vi "Conf Temp.vi"(8 "error in (no error)":errorcluster, 11 "IncTemperature":T1={"ConnectedTempSensor"="100", "ConvertMode"="1", "InitGainSelection"="0", "FrequencySelection"="240", "PowerSaveMode"=FALSE, "GainSelection"="", "RefValue"=0.0}) -> (0 "error out":errorcluster, 3 "IncTemperature Out":T1={"ConnectedTempSensor"="500", "ConvertMode"="1", "InitGainSelection"="32", "FrequencySelection"="240 Hz", "PowerSaveMode"=FALSE, "GainSelection"="", "RefValue"=0.0})   [LabVIEW 2014, in "MSX-E3711_dll.lvlib"]
uses:
  MSX-E3711_dll.lvlib
panel:
  in  "Frecuencia":string(combo)="240 Hz"
  in  "Ganancia":string(combo)="0"
  in  "Unidad":string(combo)="1"
  in  "Tipo de Sensor":string(combo)="1000"
  in  "Cancelar":bool
  in  "Save Button":bool
  # "Configurar Temperatura"
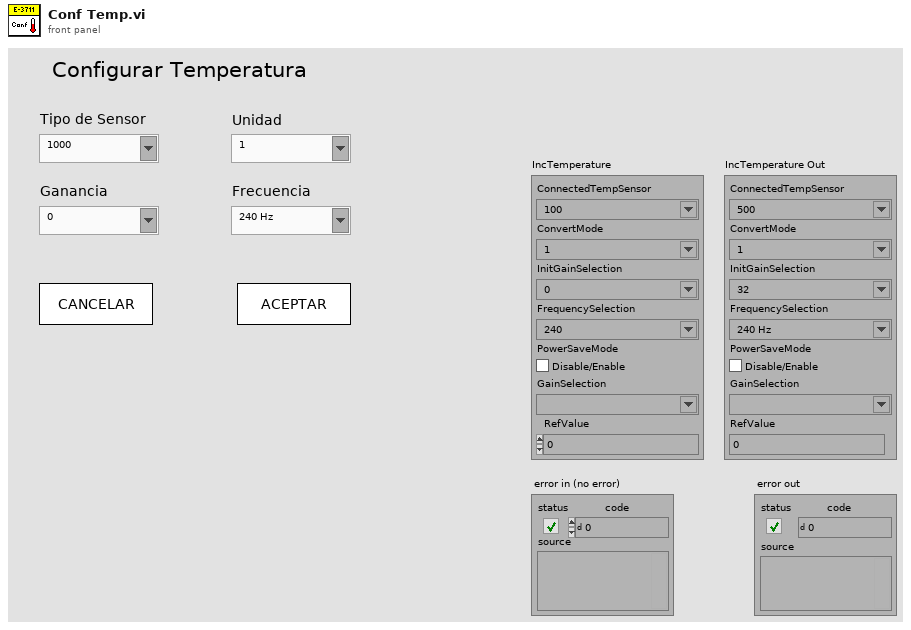
[diagram p1: front panel]
types:
  T1 = cluster{"ConnectedTempSensor":string, "ConvertMode":string, "InitGainSelection":string, "FrequencySelection":string, "PowerSaveMode":bool, "GainSelection":string, "RefValue":dbl}
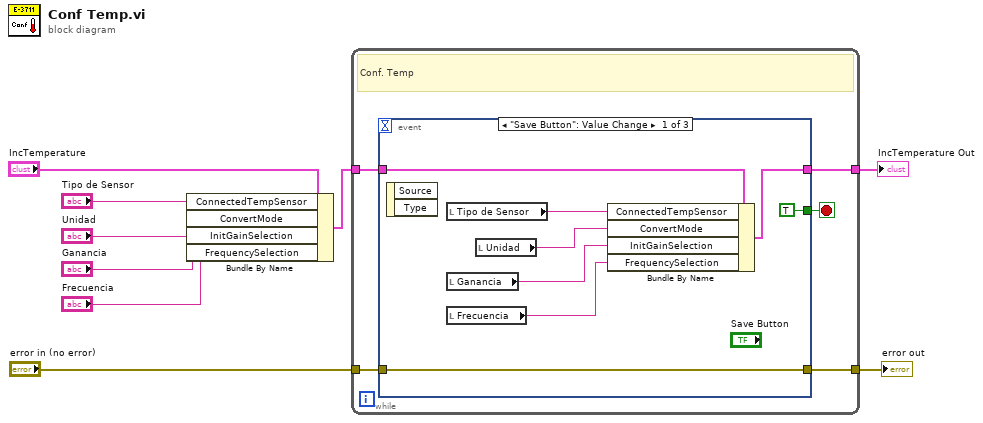
[diagram p0: block diagram]
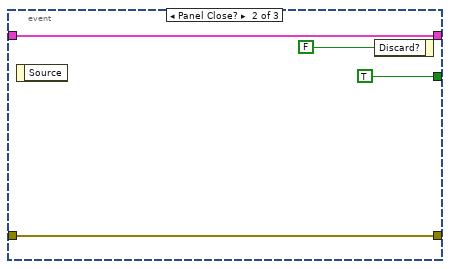
[diagram p2: hidden frame]
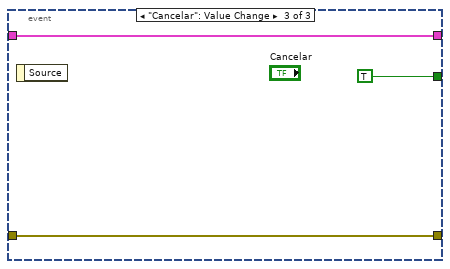
[diagram p3: hidden frame]
diagram:
  n1 = Bundle By Name(cluster="IncTemperature", "ConnectedTempSensor"="Tipo de Sensor", "ConvertMode"="Unidad", "InitGainSelection"="Ganancia", "FrequencySelection"="Frecuencia") -> (w5:T1)
  n2 = while {
    tunnel: [w13] -> w9
    tunnel: w5 -> [w12]
    tunnel: "error in (no error)" -> [w11]
    tunnel: [w10] -> w7
    stop <- w14 stop-if-true
    # "Conf. Temp"
    n3 = event shown="[0] \"Save Button\": Value Change" {
      selector: _ -> [_ _ _]
      dyn-events: _ -> [_ _ _]
      timeout: _ -> [_ _ _]
      tunnel: [TRUE ("Save Button") TRUE ("Save Button") TRUE ("Save Button")] -> w14
      tunnel: [w19 w24 w28] -> w13
      tunnel: w12 -> [w20 w24 w28]
      tunnel: w11 -> [w21 w23 w27]
      tunnel: [w21 w23 w27] -> w10
      event "Save Button": Value Change {
        n4 = event-data() -> ()  [unwired: 1 in, 2 out]
        n5 = local read "Tipo de Sensor"() -> (w18:string)
        n6 = local read "Ganancia"() -> (w16:string)
        n7 = local read "Frecuencia"() -> (w15:string)
        n8 = local read "Unidad"() -> (w17:string)
        n9 = Bundle By Name(cluster=w20, "ConnectedTempSensor"=w18, "ConvertMode"=w17, "InitGainSelection"=w16, "FrequencySelection"=w15) -> (w19:T1)
      }
      event Panel Close? {
        n10 = event-data() -> ()  [unwired: 1 in, 1 out]
        n11 = event-data("Discard?"=FALSE) -> ()  [unwired: 1 in, 1 out]
      }
      event "Cancelar": Value Change {
        n12 = event-data() -> ()  [unwired: 1 in, 1 out]
      }
    }
  }
  "error out" <- w7
  "IncTemperature Out" <- w9
